vi "Letter to Index.vi"(1 "String":string) -> (0 "Index":i32)   [LabVIEW 2020, in "Control Experiment.lvclass"]
uses:
  Control Experiment.lvclass
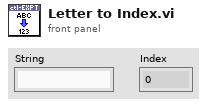
[diagram p1: front panel]
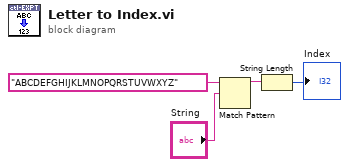
[diagram p0: block diagram]
diagram:
  n1 = Match Pattern(string="ABCDEFGHIJKLMNOPQRSTUVWXYZ", regular expression="String") -> (before substring=w2:string)  [unwired: 1 in, 3 out]
  n2 = String Length(string=w2) -> (length=→"Index":i32)
